vi "under revision Chroma 1905x Series Memory Save.vi"(8 "error in (no error)":errorcluster, 9 "Name":string, 10 "Memory Location":u32=1 min=1 max=99, 11 "inst handle in":refnum<visa-resource-name>) -> (0 "error out 2":errorcluster, 3 "inst handle out":refnum<visa-resource-name>)   [LabVIEW 2025]
doc: "Chroma\n5 Clock Tower Place Suite 210\nMaynard, MA 01754\nTel: 1 800 253-1230\nTel: 1 877 4 A HIPOT\nFax: 1 978-461-4295\nWebsite: www.chroma.com"
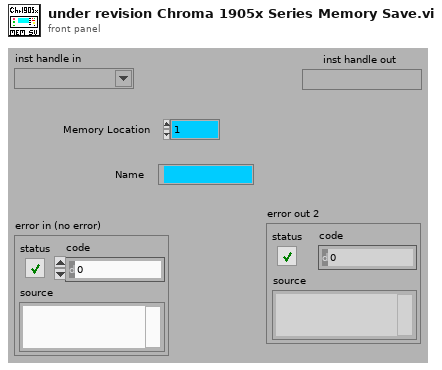
[diagram p1: front panel]
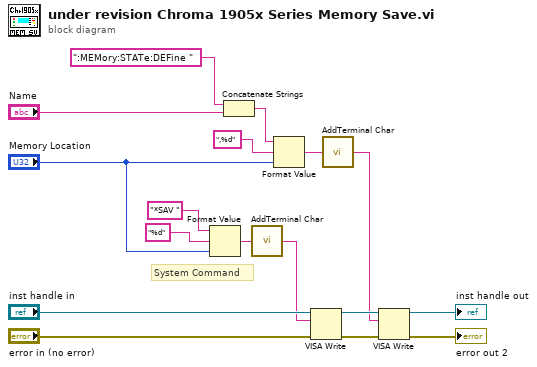
[diagram p0: block diagram]
diagram:
  # "System Command"
  n1 = Format Value(string ("")="*SAV ", format string="%d", value (0)="Memory Location") -> (output string=w6:string)
  n2 = Concatenate Strings(":MEMory:STATe:DEFine ", "Name") -> (w13:string)
  n3 = call "AddTerminal Char.vi"("Cmd string"=w6) -> ("Concatenated String"=w5:string)  [unwired: 4 in]
  n4 = Format Value(string ("")=w13, format string=",%d", value (0)="Memory Location") -> (output string=w3:string)
  n5 = VISA Write(VISA resource name="inst handle in", write buffer=w5, error in (no error)="error in (no error)") -> (VISA resource name out=w10:refnum<visa-resource-name>, error out=w11:errorcluster)  [unwired: 1 out]
  n6 = call "AddTerminal Char.vi"("Cmd string"=w3) -> ("Concatenated String"=w4:string)  [unwired: 4 in]
  n7 = VISA Write(VISA resource name=w10, write buffer=w4, error in (no error)=w11) -> (VISA resource name out=→"inst handle out":refnum<visa-resource-name>, error out=→"error out 2":errorcluster)  [unwired: 1 out]
